vi "ws_verify user login.vi"(6 "Required Permisions":T2, 7 "httpRequestID":u32, 9 "Force Authorization? (f)":bool, 10 "Logout? (f)":bool) -> (0 "error out":errorcluster, 1 "User Verified\nand Spartan\nAuthorized?":bool, 3 "DB Connection Ref":T1, 4 "User":T2)   [LabVIEW 2011]
uses:
  server/database/Users/User Record.ctl
  SI.LIB/ODBC/SQL Controls/Connection Refnum.ctl
  <vilib>/wsapi/NI_WebServices.lvlib
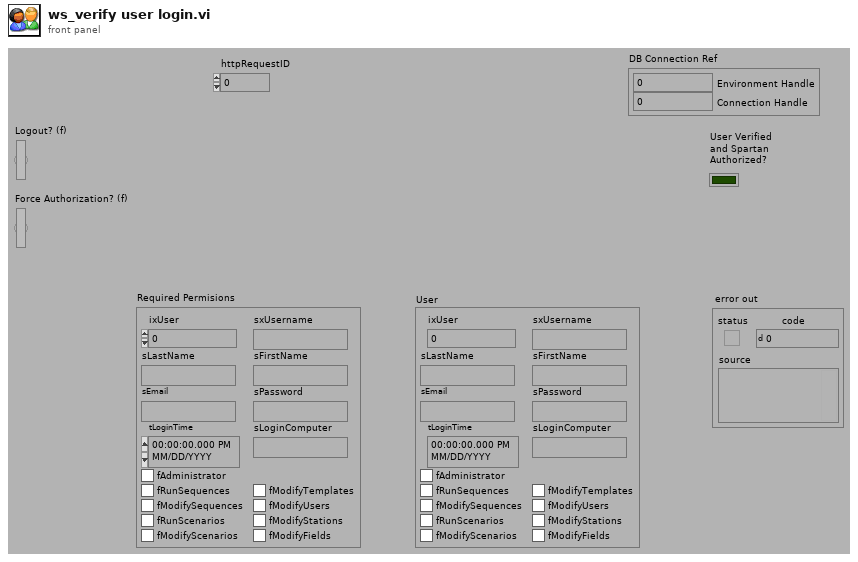
[diagram p1: front panel]
types:
  T1 = typedef "Connection Refnum.ctl" = cluster{"Environment Handle":i32, "Connection Handle":i32}
  T2 = typedef "User Record.ctl" = cluster{"ixUser":i32, "sxUsername":string, "sLastName":string, "sFirstName":string, "sEmail":string, "sPassword":string, "tLoginTime":timestamp, "sLoginComputer":string, "fAdministrator":bool, "fRunSequences":bool, "fModifySequences":bool, "fRunScenarios":bool, "fModifyScenarios":bool, "fModifyTemplates":bool, "fModifyUsers":bool, "fModifyStations":bool, "fModifyFields":bool}
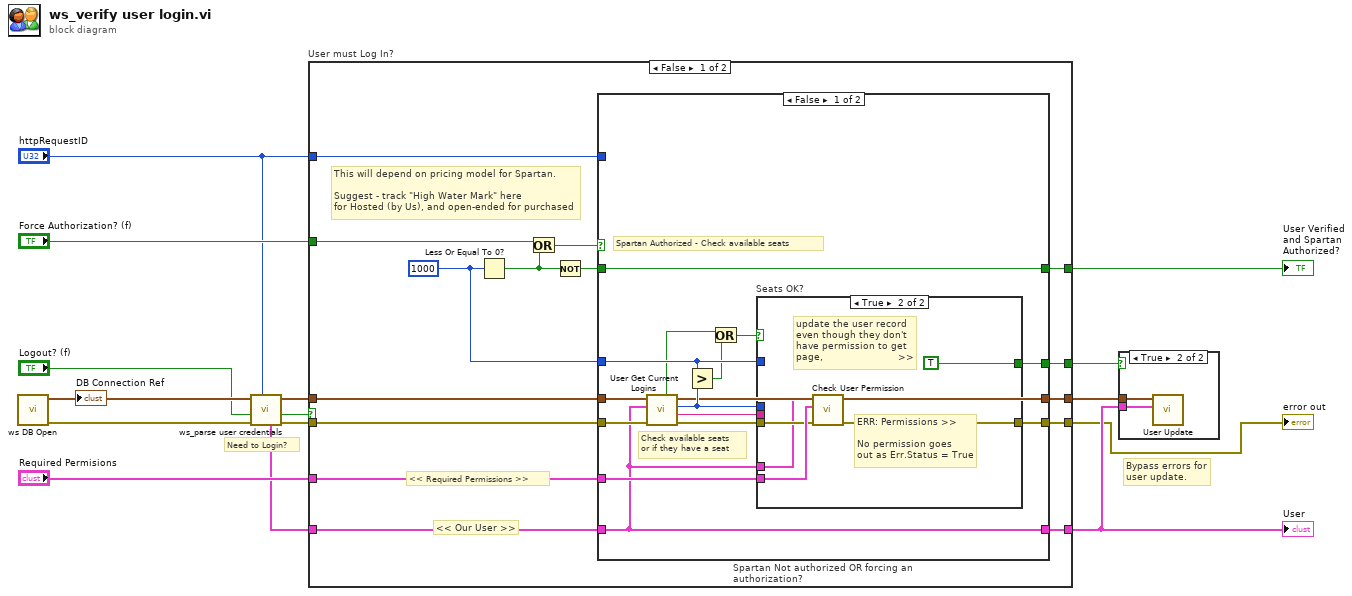
[diagram p0: block diagram]
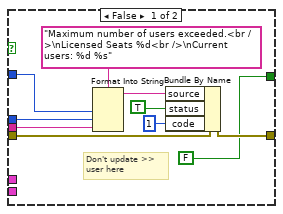
[diagram p3: hidden frame]
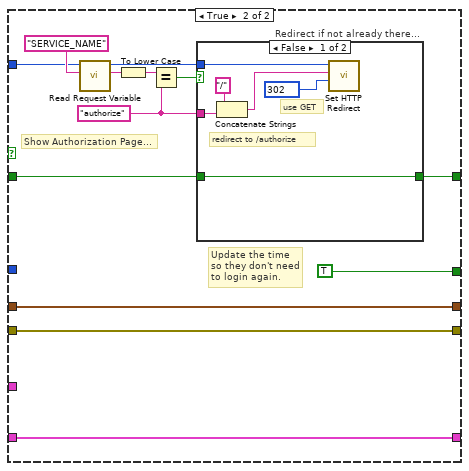
[diagram p4: hidden frame]
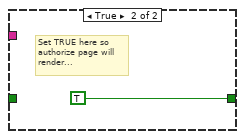
[diagram p5: hidden frame]
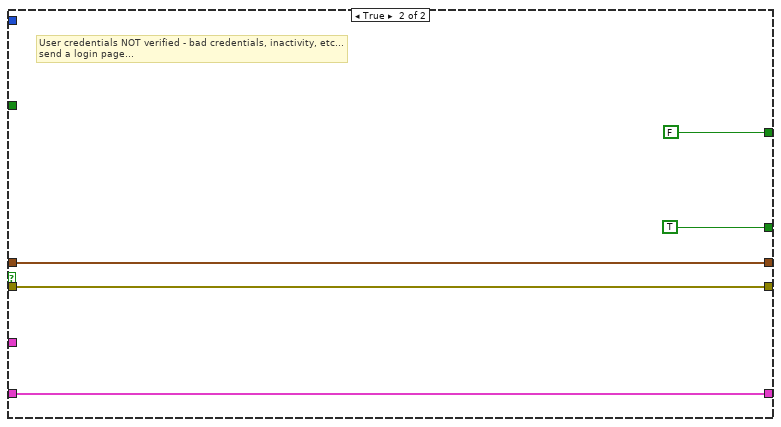
[diagram p6: hidden frame]
diagram:
  # "Bypass errors for\nuser update."
  # "Need to Login?"
  n1 = call "ws DB Open.vi"() -> ("error out"=w6:errorcluster, "Connection Refnum"=w5:T1)  [unwired: 10 in]
  "DB Connection Ref" <- w5
  n2 = call "ws_parse user credentials.vi"("httpRequestID"="httpRequestID", "error in (no error)"=w6, "Force Logout? (f)"="Logout? (f)", "DB Connection Ref"=w5) -> ("error out"=w12:errorcluster, "Login?"=w13:bool, "dup DB Connection Ref"=w11:T1, "User"=w1:T2)  [unwired: 4 in]
  n3 = case "User must Log In?" shown="False" w13 {
    tunnel: [w30 w81] -> w7
    tunnel: w12 -> [w17 w81]
    tunnel: [w22 FALSE] -> w14
    tunnel: "Required Permisions" -> [w29 _]
    tunnel: w1 -> [w28 w84]
    tunnel: [w27 w84] -> w8
    tunnel: w11 -> [w25 w82]
    tunnel: [w24 w82] -> w10
    tunnel: [w20 TRUE] -> w9
    tunnel: "Force Authorization? (f)" -> [w19 _]
    tunnel: "httpRequestID" -> [w18 _]
    frame False {
      w16 = 1000
      # "This will depend on pricing model for Spartan.\n\nSuggest - track \"High Water Mark\" here\nfor Hosted (by Us), and open-ended for purchased"
      # "<< Our User >>"
      # "<< Required Permissions >>"
      n4 = Less Or Equal To 0?(x=w16) -> (x <= 0?=w21:bool)
      n5 = Or(x=w19, y=w21) -> (x .or. y?=w26:bool)
      n6 = Not(x=w21) -> (.not. x?=w23:bool)
      n7 = case "Spartan Not authorized OR forcing an authorization?" shown="False" w26 {
        tunnel: w17 -> [w43 w61]
        tunnel: [w45 w61] -> w30
        tunnel: w29 -> [w44 _]
        tunnel: w28 -> [w37 w73]
        tunnel: [w37 w73] -> w27
        tunnel: w25 -> [w38 w65]
        tunnel: [w31 w65] -> w24
        tunnel: w23 -> [w40 w68]
        tunnel: [w40 w67] -> w22
        tunnel: w16 -> [w39 _]
        tunnel: [w32 TRUE] -> w20
        tunnel: w18 -> [_ w63]
        frame False {
          # "Spartan Authorized - Check available seats"
          # "Check available seats\nor if they have a seat"
          n8 = call "User Get Current Logins.vi"("error in (no error)"=w43, "Current User (none)"=w37, "Connection Refnum"=w38) -> ("error out"=w42:errorcluster, "Current User Summary"=w36:string, "Seats in Use"=w35:i32, "dup Connection Refnum"=w31:T1, "Current User has Seat?"=w34:bool)  [unwired: 1 in, 3 out]
          n9 = Greater?(x=w39, y=w35) -> (0:w33:bool)
          n10 = Or(x=w34, y=w33) -> (x .or. y?=w41:bool)
          n11 = case "Seats OK?" shown="True" w41 {
            tunnel: [w51 w57] -> w45
            tunnel: w44 -> [_ w60]
            tunnel: w42 -> [w48 w59]
            tunnel: w39 -> [w55 _]
            tunnel: w37 -> [_ w58]
            tunnel: w35 -> [w53 _]
            tunnel: w36 -> [w50 _]
            tunnel: [FALSE TRUE] -> w32
            frame False {
              # "Don't update >>\nuser here"
              n12 = Format Into String(format string="Maximum number of users exceeded.<br />\nLicensed Seats %d<br />\nCurrent users: %d %s", w55, w53, w50) -> (resulting string=w52:string)  [unwired: 2 in, 1 out]
              n13 = Bundle By Name(cluster=w48, "source"=w52, "status"=TRUE, "code"=1) -> (w51:errorcluster)
            }
            frame True {
              # "update the user record\neven though they don't\nhave permission to get\npage,                         >>"
              # "ERR: Permissions >>\n\nNo permission goes\nout as Err.Status = True"
              n14 = call "Check User Permission.vi"("error in"=w59, "Required Permisions"=w60, "User Record"=w58) -> ("error out"=w57:errorcluster)  [unwired: 8 out]
            }
          }
        }
        frame True {
          w70 = "authorize" ("New URL (/cgi-bin/testing.vit)")
          # "Update the time\nso they don't need\nto login again."
          # "Show Authorization Page..."
          n15 = call <vilib>:"Read Request Variable.vi"("variable name"="SERVICE_NAME" ("New URL (/cgi-bin/testing.vit)"), "httpRequestID"=w63) -> ("value"=w71:string, "httpRequestID out"=w62:u32)  [unwired: 7 in, 1 out]
          n16 = To Lower Case(string=w71) -> (all lower case string=w66:string)
          n17 = Equal?(x=w66, y=w70) -> (x = y?=w69:bool)
          n18 = case "Redirect if not already there..." shown="False" w69 {
            tunnel: w70 -> [w77 _]
            tunnel: w68 -> [w79 _]
            tunnel: [w79 TRUE] -> w67
            tunnel: w62 -> [w78 _]
            frame False {
              w74 = 302 items=["100"=100, "101"=101, "200"=200, "201"=201, "202"=202, "203"=203, "204"=204, "205"=205, "206"=206, "300"=300, "301"=301, "302"=302, "303"=303, "304"=304, "305"=305, "306"=306, "307"=307, "400"=400, "401"=401, "402"=402, "403"=403, "404"=404, "405"=405, "406"=406, "407"=407, "408"=408, "409"=409, "410"=410, "411"=411, "412"=412, "413"=413, "414"=414, "415"=415, "416"=416, "417"=417, "500"=500, "501"=501, "502"=502, "503"=503, "504"=504, "505"=505] ("response code (307)")
              # "use GET"
              # "redirect to /authorize"
              n19 = Concatenate Strings("/" ("New URL (/cgi-bin/testing.vit)"), w77) -> (w76:string)
              n20 = call <vilib>:"Set HTTP Redirect.vi"("response code (307)"=w74, "redirect URL"=w76, "httpRequestID"=w78) -> ()  [unwired: 7 in, 2 out]
            }
            frame True {
              # "Set TRUE here so\nauthorize page will\nrender..."
            }
          }
        }
      }
    }
    frame True {
      # "User credentials NOT verified - bad credentials, inactivity, etc...\nsend a login page..."
    }
  }
  "error out" <- w7
  "User Verified\nand Spartan\nAuthorized?" <- w14
  "User" <- w8
  n21 = case shown="True" w9 {
    tunnel: w10 -> [_ w87]
    tunnel: w8 -> [_ w86]
    frame False {
    }
    frame True {
      n22 = call "User Update.vi"("User Record"=w86, "Connection Refnum"=w87) -> ()  [unwired: 1 in, 9 out]
    }
  }
